vi "Power Nominal Write Single.vi"(8 "error in":errorcluster, 9 "Channel Index":i32=1, 10 "Power Nominal AV":dbl, 11 "Cycler in":refnum<class "Cycler.lvclass">) -> (0 "error out":errorcluster, 3 "Cycler out":refnum<class "Cycler.lvclass">)   [LabVIEW 2023, in "Cycler.lvclass"]
uses:
  Cycler.lvclass
  Cycler.lvclass/Cycler.ctl
  Low Level Capabilities/Power/Power Nominal Value/Power Nominal Value.lvclass
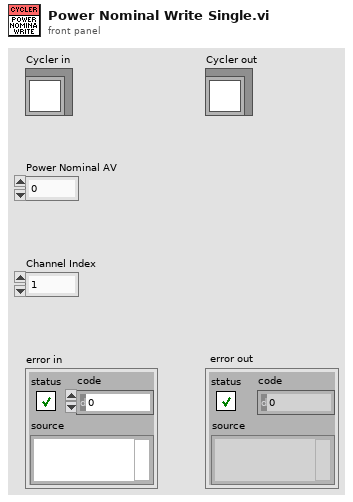
[diagram p1: front panel]
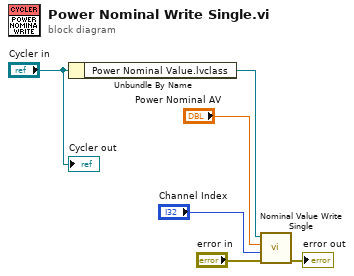
[diagram p0: block diagram]
diagram:
  n1 = Unbundle By Name("Cycler in") -> ("Power Nominal Value.lvclass"=w5:refnum<class "Power Nominal Value.lvclass">)
  n2 = call-dynamic "Nominal Value Write Single.vi"("error in"="error in", "Channel Index"="Channel Index", "Power Nominal Value"="Power Nominal AV", "Power Nominal Value in"=w5) -> ("error out"=→"error out":errorcluster)  [unwired: 6 in, 1 out]
  "Cycler out" <- "Cycler in"
